vi "GetCXT.vi"(5 "format string (%.;%_20f)":string="%.;%_20f", 7 "key description":string, 8 "sections":string[](array[string]), 9 "numeric":cxt, 11 "info data":string) -> (0 "sections out":string[](array[string]), 1 "key found?":bool, 2 "value":cxt format="%#_20g", 3 "info data out":string)   [LabVIEW 2020, in "infolib.lvlib"]
doc: "Add a new numeric key to Info Data string. If section exists in Info Data string, inserts key into this section."
uses:
  infolib.lvlib
panel:
  out "value 3":ext
  out "value 2":ext
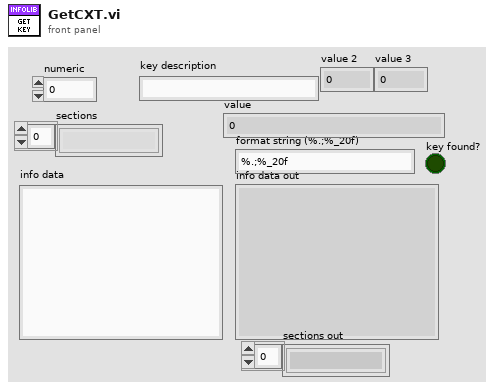
[diagram p1: front panel]
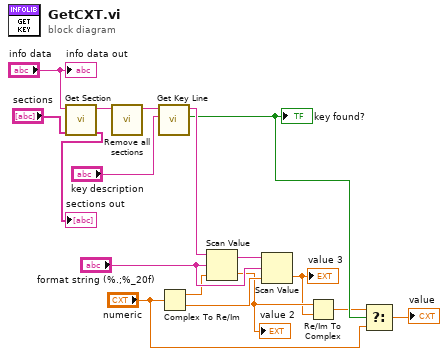
[diagram p0: block diagram]
diagram:
  n1 = call "Get Section.vi"("sections"="sections", "info data"="info data") -> ("sections out"=→"sections out":string[], "section part"=w17:string)  [unwired: 7 in, 1 out]
  n2 = call "Remove all sections.vi"("info data"=w17) -> ("info data out"=w16:string)  [unwired: 10 in]
  n3 = call "Get Key Line.vi"("key description"="key description", "info data"=w16) -> ("key found?"=w4:bool, "key value"=w13:string)  [unwired: 8 in]
  "key found?" <- w4
  n4 = Complex To Re/Im(x + iy="numeric") -> (x=w10:ext, y=w9:ext)
  n5 = Scan Value(string=w13, format string="format string (%.;%_20f)", default (0 dbl)=w10) -> (output string=w12:string, value=w8:ext)
  "value 2" <- w8
  n6 = Scan Value(string=w12, format string="format string (%.;%_20f)", default (0 dbl)=w9) -> (value=w7:ext)  [unwired: 1 out]
  "value 3" <- w7
  n7 = Re/Im To Complex(1:w7, 2:w8) -> (0:w1:cxt)
  n8 = Select(t=w1, s=w4, f="numeric") -> (s? t:f=→"value":cxt)
  "info data out" <- "info data"
